vi "SUB_COM_W_CharByCharNoCarrige_chkstring.vi"(2 "cmd string":string, 3 "duplicate VISA resource name":refnum<visa-resource-name>) -> (0 "OUT string":string, 1 "VISA resource OUT":refnum<visa-resource-name>)   [LabVIEW 2011]
panel:
  out "out1":string
  out "LOOP":i32
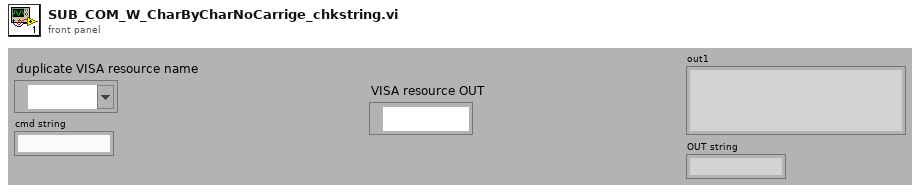
[diagram p1: front panel]
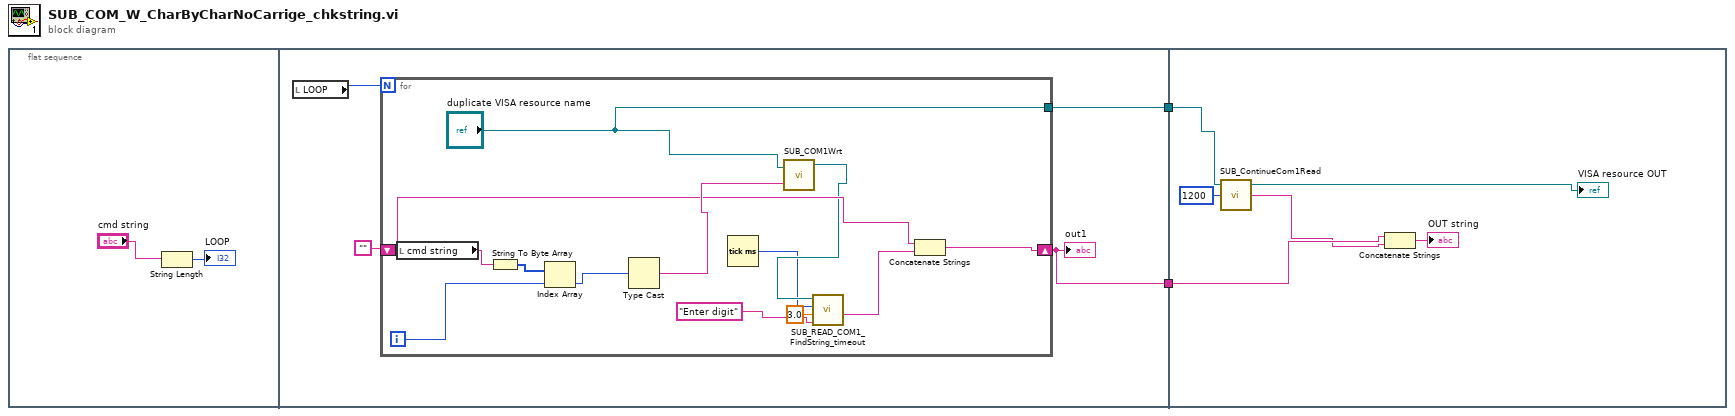
[diagram p0: block diagram]
diagram:
  n1 = flat-sequence {
    tunnel: [w7] -> w2
    tunnel: [w5] -> w1
    tunnel: w2 -> [w26]
    tunnel: w1 -> [w24]
    frame #0 {
      n2 = String Length(string="cmd string") -> (length=→"LOOP":i32)
    }
    frame #1 {
      n3 = local read "LOOP"() -> (w8:i32)
      n4 = for {
        N: w8 -> [_]
        tunnel: ["duplicate VISA resource name"] -> w7
        shift-right: [w16] -> w5
        shift-left: "" -> [w15]
        i -> [w19]
        n5 = local read "cmd string"() -> (w21:string)
        n6 = String To Byte Array(string=w21) -> (unsigned byte array=w20:u8[])
        n7 = Index Array(array=w20, index=w19) -> (element=w18:u8)
        n8 = Type Cast(x=w18) -> (*(type *) &x=w17:string)  [unwired: 1 in]
        n9 = Tick Count (ms)() -> (millisecond timer value=w11:u32)
        n10 = call "SUB_COM1Wrt.vi"("VISA resource name"="duplicate VISA resource name", "write buffer"=w17) -> ("duplicate VISA resource name"=w12:refnum<visa-resource-name>)  [unwired: 2 out]
        n11 = call "SUB_READ_COM1_FindString_timeout.vi"("Find this String"="Enter digit", "Timeout Seccond"=3.0, "Begin time"=w11, "duplicate VISA resource name 2"=w12) -> ("Output String"=w9:string)  [unwired: 1 in, 2 out]
        n12 = Concatenate Strings(w15, w9) -> (w16:string)
      }
      "out1" <- w5
    }
    frame #2 {
      n13 = call "SUB_ContinueCom1Read.vi"("Numeric"=1200, "duplicate VISA resource name 2"=w26) -> ("String"=w23:string, "duplicate VISA resource name"=→"VISA resource OUT":refnum<visa-resource-name>)  [unwired: 1 in, 1 out]
      n14 = Concatenate Strings(w24, w23) -> (→"OUT string":string)
    }
  }
